vi "Tidal Eng-Initialization.vi"(8 "error in (no error)":errorcluster, 10 "Remote Port":u16, 11 "IP Address":string) -> (0 "error out":errorcluster, 3 "Modbus Master out":refnum<class "Modbus Master.lvclass">)   [LabVIEW 2023]
uses:
  <vilib>/NI/Modbus Library/API/Master/Modbus Master.lvclass
  <vilib>/NI/Modbus Library/API/Wrapper/Create TCP Master.vi
  <vilib>/NI/Modbus Library/API/Wrapper/API Main.lvlib
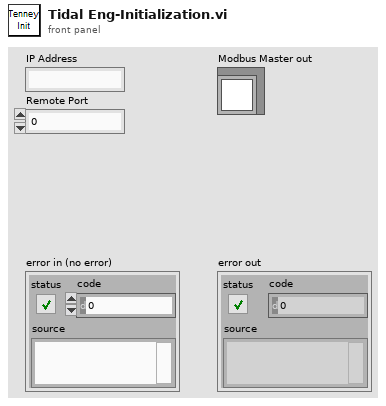
[diagram p1: front panel]
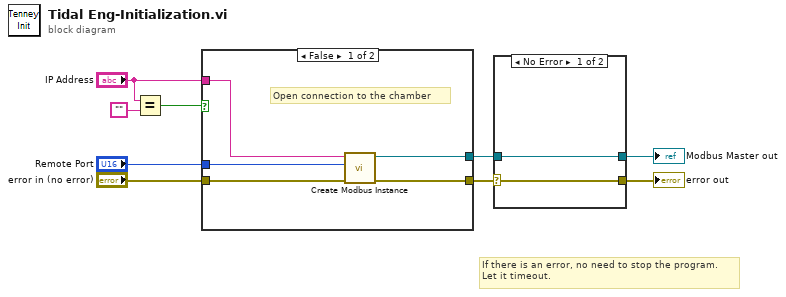
[diagram p0: block diagram]
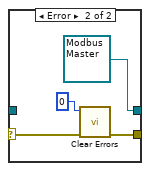
[diagram p2: hidden frame]
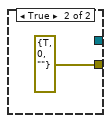
[diagram p3: hidden frame]
diagram:
  # "If there is an error, no need to stop the program. \nLet it timeout."
  n1 = Equal?(x="IP Address", y="") -> (x = y?=w5:bool)
  n2 = case shown="False" w5 {
    tunnel: [w14 _] -> w4
    tunnel: "Remote Port" -> [w13 _]
    tunnel: [w12 errorcluster {"status"=TRUE, "code"=0, "source"=""} ("error out")] -> w3
    tunnel: "error in (no error)" -> [w11 _]
    tunnel: "IP Address" -> [w10 _]
    frame False {
      # "Open connection to the chamber"
      n3 = call-poly <vilib>:"Create Modbus Instance.vi"("error in"=w11, "port (502)"=w13, "address"=w10) -> ("error out"=w12:errorcluster, "TCP master instance"=w14:refnum<class "Modbus Master.lvclass">)  [unwired: 7 in]
    }
    frame True {
    }
  }
  n4 = case shown="No Error" w3 {
    selector: w3 -> [w16 w20]
    tunnel: w4 -> [w17 _]
    tunnel: [w17 refnum<class "Modbus Master.lvclass"> refnum ("TCP master instance")] -> w2
    tunnel: [w16 w19] -> w1
    frame No Error {
    }
    frame Error {
      n5 = call <vilib>:"Clear Errors.vi"("error in (no error)"=w20, "specific error code to clear (0: all)"=0) -> ("error out"=w19:errorcluster)  [unwired: 4 in, 1 out]
    }
  }
  "Modbus Master out" <- w2
  "error out" <- w1
